vi "Reset USB&temp v 1.vi"(7 "Test":bool=TRUE) -> (0 "Reset Error":bool)   [LabVIEW 2017]
uses:
  <vilib>/Platform/TimedLoop/XDataNode/timing_clust.ctl
  <vilib>/Platform/TimedLoop/XDataNode/nitl_modes.ctl
  <vilib>/Platform/TimedLoop/XDataNode/wakeup.ctl
  <vilib>/platform/TimedLoop/XDataNode/XDataNode.xnode
  <vilib>/Platform/TimedLoop/XDataNode/XDNodeRunTimeDep.lvlib
panel:
  out "Reset Time Out":dbl
  out "Message":string
  in  "End Reset Routine":bool
  # "RESET USB $ TEMP"
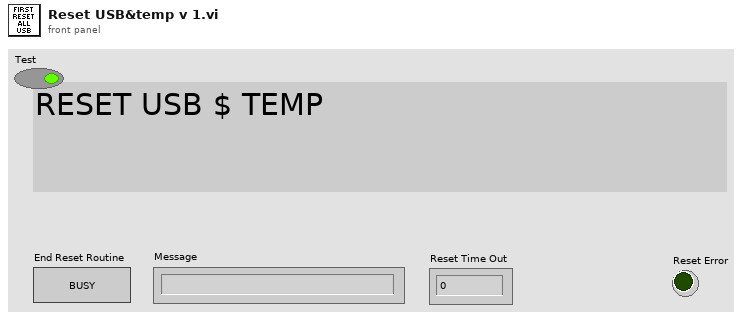
[diagram p1: front panel]
types:
  T1 = typedef "XDNodeRunTimeDep.lvlib/timing_clust.ctl" = cluster{"Expected End [f-1]":u64, "Actual End [f-1]":u64, "Finished Late? [f-1]":bool, "Expected End [i-1]":u64, "Actual End [i-1]":u64, "Finished Late? [i-1]":bool, "Expected Start [i]":u64, "Actual Start [i]":u64, "Expected Start [f]":u64, "Actual Start [f]":u64, "Source Name":string, "Structure Name":string, "Period":i64, "Deadline":i64, "Offset":i64, "Start":i64, "Priority":i32, "Timeout":i32, "Mode":T2, "Wakeup Reason":T3, "Error":errorcluster, "Source Type":string, "Secondary Source Type":string, "Global End Time":u64, "Global Start Time":u64, "Frame Duration":u64, "Iteration Duration":u64, "Assigned CPU":i32, "I/O Scan Engine Mode":u32}
  T2 = typedef "XDNodeRunTimeDep.lvlib/nitl_modes.ctl" = enum32{"No Change", "Process missed periods, maintain original phase", "Discard missed periods, maintain original phase", "Process missed periods, ignore original phase", "Discard missed periods, ignore original phase"}
  T3 = typedef "XDNodeRunTimeDep.lvlib/wakeup.ctl" = enum32{"Normal", "Aborted", "Asynchronous wakeup", "Timing source error", "Timed loop error", "Timeout"}
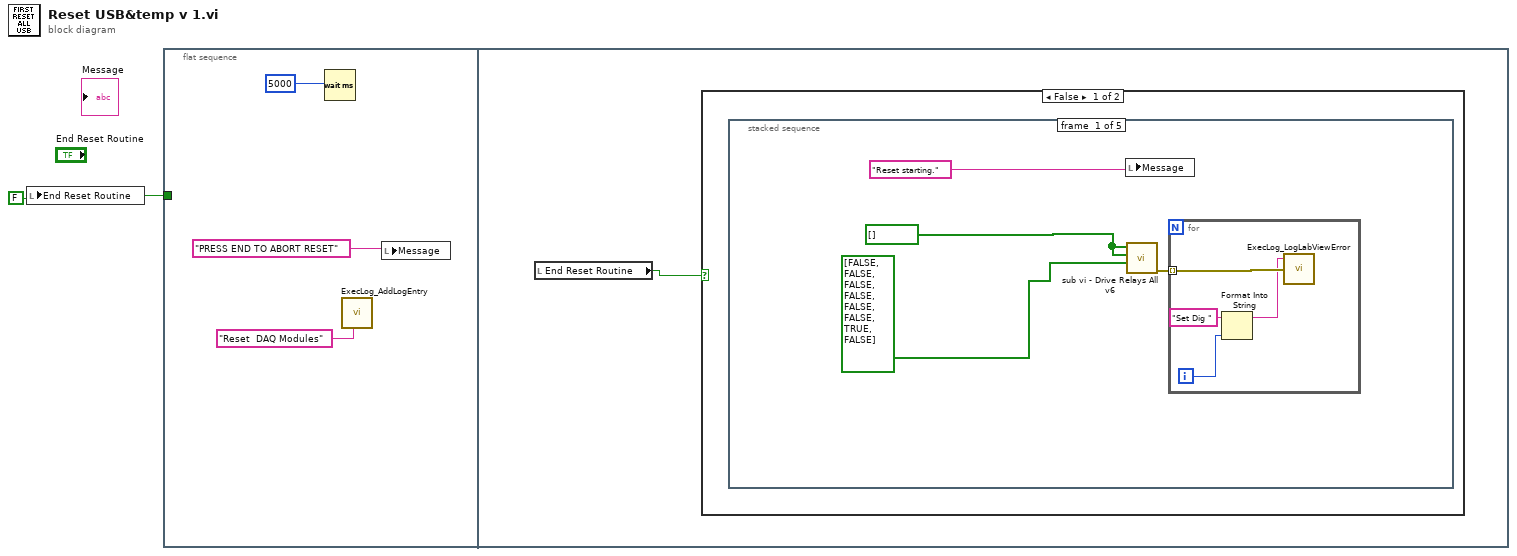
[diagram p0: block diagram]
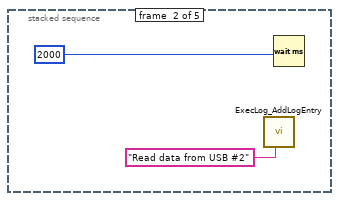
[diagram p2: hidden frame]
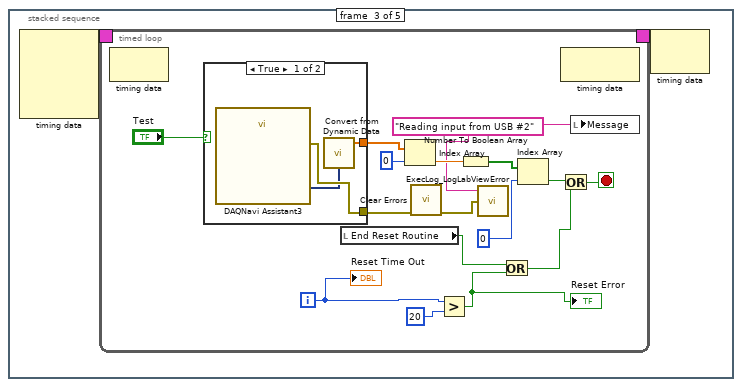
[diagram p3: hidden frame]
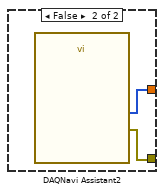
[diagram p4: hidden frame]
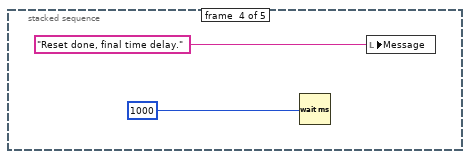
[diagram p5: hidden frame]
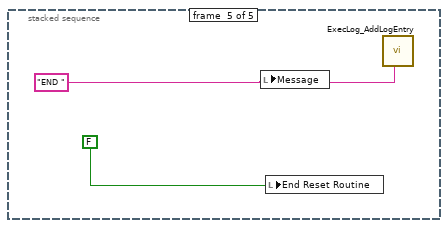
[diagram p6: hidden frame]
diagram:
  w1 = FALSE
  n1 = local write "End Reset Routine"(w1) -> ()
  n2 = flat-sequence {
    tunnel: w1 -> [_]
    frame #0 {
      n3 = Wait (ms)(milliseconds to wait=5000) -> ()  [unwired: 1 out]
      n4 = call "ExecLog_AddLogEntry.vi"("Msg"="Reset  DAQ Modules") -> ()  [unwired: 7 in, 3 out]
      n5 = local write "Message"("PRESS END TO ABORT RESET") -> ()
    }
    frame #1 {
      n6 = local read "End Reset Routine"() -> (w5:bool)
      n7 = case shown="False" w5 {
        frame False {
          n8 = stacked-sequence {
            frame #0 {
              w8 = bool[] []
              n9 = local write "Message"("Reset starting.") -> ()
              n10 = call "sub vi - Drive Relays All v6.vi"("Array #2"=bool[] [FALSE, FALSE, FALSE, FALSE, FALSE, FALSE, TRUE, FALSE], "Array #1"=w8, "Array #0"=w8) -> ("error Array"=w6:errorcluster[])  [unwired: 8 in]
              n11 = for {
                tunnel: w6 -> [w13] mode=indexing
                i -> [w11]
                n12 = Format Into String(initial string="Set Dig ", w11) -> (resulting string=w10:string)  [unwired: 2 in, 1 out]
                n13 = call "ExecLog_LogLabViewError.vi"("error IO"=w13, "string 1"=w10) -> ()  [unwired: 2 in, 1 out]
              }
            }
            frame #1 {
              n14 = call "ExecLog_AddLogEntry.vi"("Msg"="Read data from USB #2") -> ()  [unwired: 7 in, 3 out]
              n15 = Wait (ms)(milliseconds to wait=2000) -> ()  [unwired: 1 out]
            }
            frame #2 {
              n16 = node-c288() -> (w17:T1)  [unwired: 4 in]
              n17 = timed-loop {
                timing: w17 -> [_]
                timing-out: [_] -> w16
                i -> [w21]
                stop <- w29 stop-if-true
                w18 = "Reading input from USB #2"
                n18 = node-c288() -> ()  [unwired: 1 in, 1 out]
                n19 = case shown="True" "Test" {
                  tunnel: [w34 w38] -> w27
                  tunnel: [w36 w37] -> w26
                  frame True {
                    n20 = call "DAQNavi Assistant3"() -> ("error out"=w36:errorcluster, "data out(DDT)"=w35:dynamicdata)  [unwired: 26 in]
                    n21 = call "Convert from Dynamic Data"("Dynamic Data Type"=w35) -> ("Array"=w34:dbl[])  [unwired: 3 in]
                  }
                  frame False {
                    n22 = call "DAQNavi Assistant2"() -> ("error out"=w37:errorcluster, "dataOut(U8Array)"=w38:u8[])  [unwired: 26 in]
                  }
                }
                n23 = local read "End Reset Routine"() -> (w25:bool)
                n24 = Index Array(array=w27, index=0) -> (element=w31:dbl)
                n25 = call <vilib>:"Clear Errors.vi"("error in (no error)"=w26) -> ("error out"=w19:errorcluster)  [unwired: 5 in, 1 out]
                n26 = Greater?(x=w21, y=20) -> (0:w22:bool)
                "Reset Error" <- w22
                n27 = Number To Boolean Array(number=w31) -> (Boolean array=w32:bool[])
                n28 = call "ExecLog_LogLabViewError.vi"("error IO"=w19, "string 1"=w18) -> ()  [unwired: 2 in, 1 out]
                n29 = Or(x=w25, y=w22) -> (x .or. y?=w23:bool)
                n30 = Index Array(array=w32, index=0) -> (element=w28:bool)
                n31 = node-c288() -> ()  [unwired: 1 in, 1 out]
                n32 = Or(x=w28, y=w23) -> (x .or. y?=w29:bool)
                n33 = local write "Message"(w18) -> ()
                "Reset Time Out" <- w21
              }
              n34 = node-c288(w16) -> ()  [unwired: 1 out]
            }
            frame #3 {
              n35 = Wait (ms)(milliseconds to wait=1000) -> ()  [unwired: 1 out]
              n36 = local write "Message"("Reset done, final time delay.") -> ()
            }
            frame #4 {
              w45 = "END "
              n37 = local write "Message"(w45) -> ()
              n38 = local write "End Reset Routine"(FALSE) -> ()
              n39 = call "ExecLog_AddLogEntry.vi"("Msg"=w45) -> ()  [unwired: 7 in, 3 out]
            }
          }
        }
        frame True {
        }
      }
    }
  }
